vi "题目3.vi"(1 "温度":string, 2 "停止":bool, 3 "温度单位":bool) -> (0 "温度计":dbl(slide) scale=0.0..200.0)   [LabVIEW 2017]
panel:
  # "°F"
  # "°C"
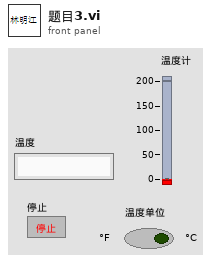
[diagram p1: front panel]
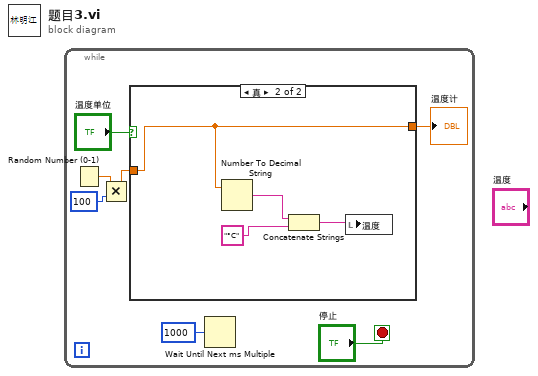
[diagram p0: block diagram]
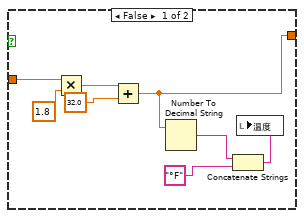
[diagram p2: hidden frame]
diagram:
  n1 = while {
    stop <- "停止" stop-if-true
    n2 = Random Number (0-1)() -> (number: 0 to 1=w5:dbl)
    n3 = Multiply(x=w5, y=100) -> (x*y=w3:dbl)
    n4 = case shown="真" "温度单位" {
      tunnel: w3 -> [w14 w17]
      tunnel: [w11 w17] -> w1
      frame False {
        n5 = Multiply(x=w14, y=1.8) -> (x*y=w13:dbl)
        n6 = Add(x=w13, y=32.0) -> (x+y=w11:dbl)
        n7 = Number To Decimal String(number=w11) -> (decimal integer string=w10:string)  [unwired: 1 in]
        n8 = Concatenate Strings(w10, "°F") -> (w8:string)
        n9 = local write "温度"(w8) -> ()
      }
      frame True {
        n10 = Number To Decimal String(number=w17) -> (decimal integer string=w19:string)  [unwired: 1 in]
        n11 = Concatenate Strings(w19, "°C") -> (w16:string)
        n12 = local write "温度"(w16) -> ()
      }
    }
    "温度计" <- w1
    n13 = Wait Until Next ms Multiple(millisecond multiple=u32 1000 ("毫秒倍数")) -> ()  [unwired: 1 out]
  }
